vi "test test.vi"(8 "error in (no error)":errorcluster, 11 "TestCase in":refnum<class "Pass If Equal Timestamp Test Case.lvclass">) -> (0 "error out":errorcluster, 3 "TestCase out":refnum<class "Pass If Equal Timestamp Test Case.lvclass">)   [LabVIEW 2015]
uses:
  Pass If Equal Timestamp Test Case.lvclass
  <vilib>/addons/_JKI Toolkits/VI Tester/TestCase.llb/TestCase.lvclass
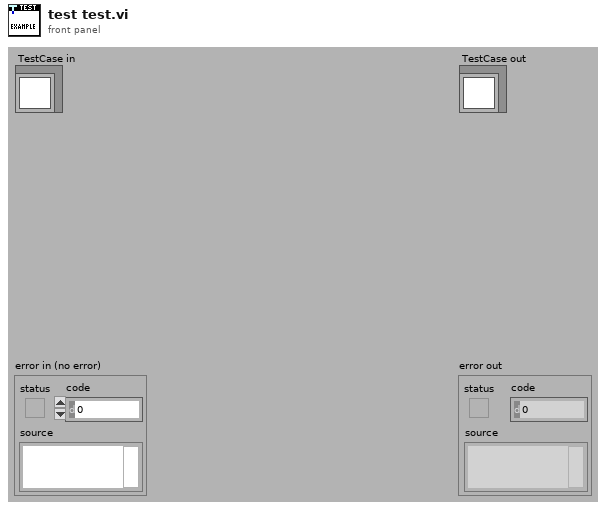
[diagram p1: front panel]
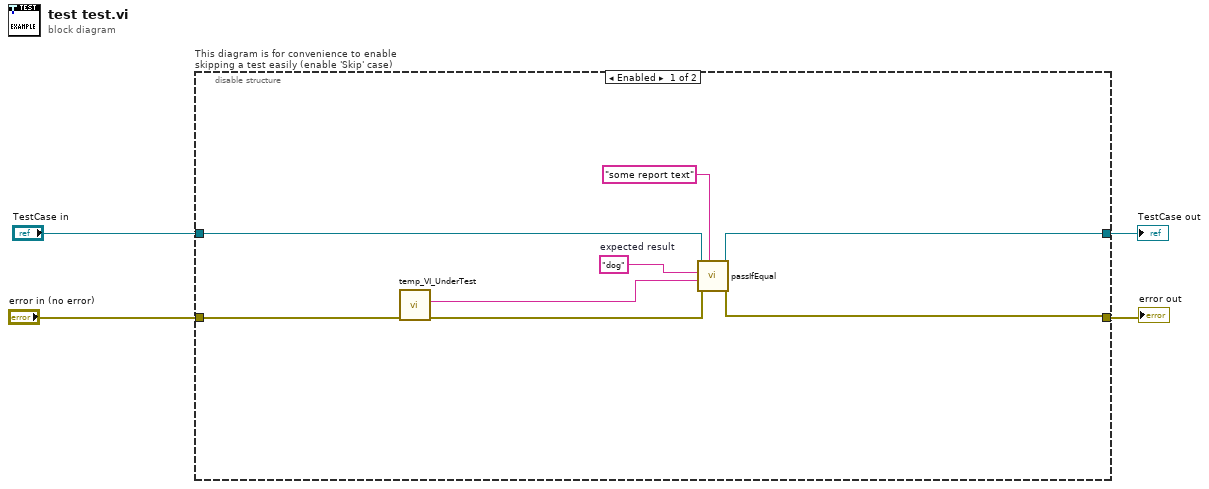
[diagram p0: block diagram]
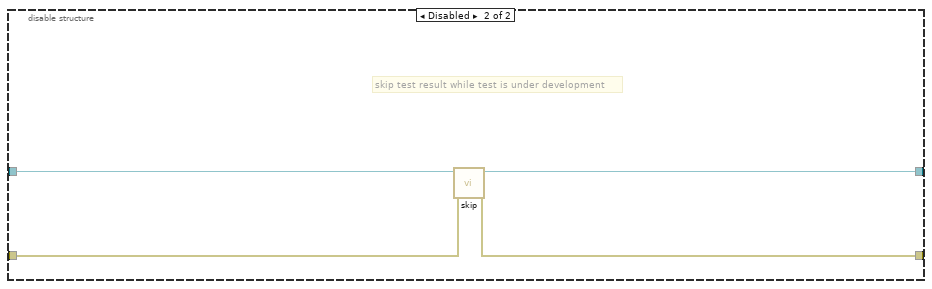
[diagram p2: hidden frame]
diagram:
  n1 = disable-structure "This diagram is for convenience to enable skipping a test easily (enable 'Skip' case)" shown="Enabled" {
    disable-tunnel: "TestCase in" -> [w11 w16]
    disable-tunnel: [w10 w14] -> w1
    disable-tunnel: [w9 w15] -> w3
    disable-tunnel: "error in (no error)" -> [w8 w13]
    frame Enabled {
      w12 = "dog"  # expected result
      n2 = call "temp_VI_UnderTest.vi"("error in"=w8) -> ("error out"=w7:errorcluster, "actual result"=w6:string)  [unwired: 9 in]
      n3 = call-dynamic "passIfEqual.vi"("custom report message (\"\")"="some report text", "error in (no error)"=w7, "y"=w6, "x"=w12, "TestCase in"=w11) -> ("error out"=w9:errorcluster, "TestCase out"=w10:refnum<class "Pass If Equal Timestamp Test Case.lvclass">)  [unwired: 5 in]
    }
    frame Disabled {
      # "skip test result while test is under development"
      n4 = call <vilib>:"skip.vi"("error in (no error)"=w13, "TestCase in"=w16) -> ("error out"=w15:errorcluster, "TestCase out"=w14:refnum<class "Pass If Equal Timestamp Test Case.lvclass">)  [unwired: 8 in]
    }
  }
  "error out" <- w3
  "TestCase out" <- w1
